vi "simulate_sine_dc.vi"(11 "Signal type":enum16{"Sine", "DC"}(ring)) -> (2 "Signal with noise":dbl[](array[numeric]), 3 "Signal":dbl[](array[numeric]))   [LabVIEW 2018]
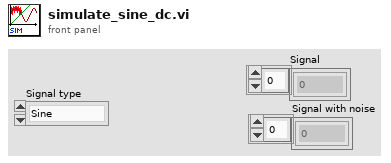
[diagram p1: front panel]
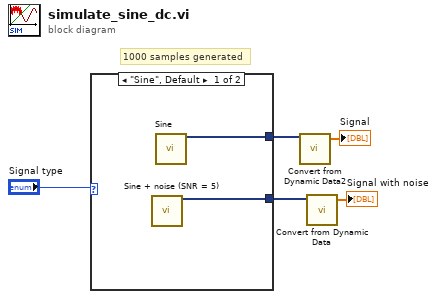
[diagram p0: block diagram]
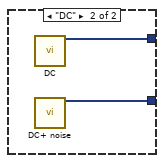
[diagram p2: hidden frame]
diagram:
  # "1000 samples generated"
  n1 = case shown="\"Sine\", Default" "Signal type" {
    tunnel: [w7 w8] -> w5
    tunnel: [w6 w9] -> w3
    frame "Sine", Default {
      n2 = call "Sine + noise (SNR = 5)"() -> ("NoisySine"=w7:dynamicdata)  [unwired: 14 in, 1 out]
      n3 = call "Sine"() -> ("Sine"=w6:dynamicdata)  [unwired: 14 in, 1 out]
    }
    frame "DC" {
      n4 = call "DC"() -> ("DC"=w9:dynamicdata)  [unwired: 14 in, 1 out]
      n5 = call "DC+ noise"() -> ("Noisy_DC"=w8:dynamicdata)  [unwired: 14 in, 1 out]
    }
  }
  n6 = call "Convert from Dynamic Data2"("Dynamic Data Type"=w3) -> ("Array"=→"Signal":dbl[])  [unwired: 3 in]
  n7 = call "Convert from Dynamic Data"("Dynamic Data Type"=w5) -> ("Array"=→"Signal with noise":dbl[])  [unwired: 3 in]
